vi "VarillaDataReadingStringToClusterFormar.vi"(11 "StringFormat":string[](array[string])) -> (3 "ClusterFormat":T1)   [LabVIEW 2014]
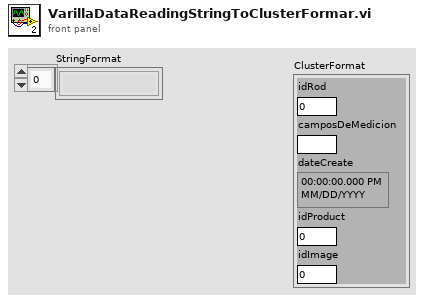
[diagram p1: front panel]
types:
  T1 = cluster{"idRod":dbl, "camposDeMedicion":string, "dateCreate":timestamp, "idProduct":dbl, "idImage":dbl}
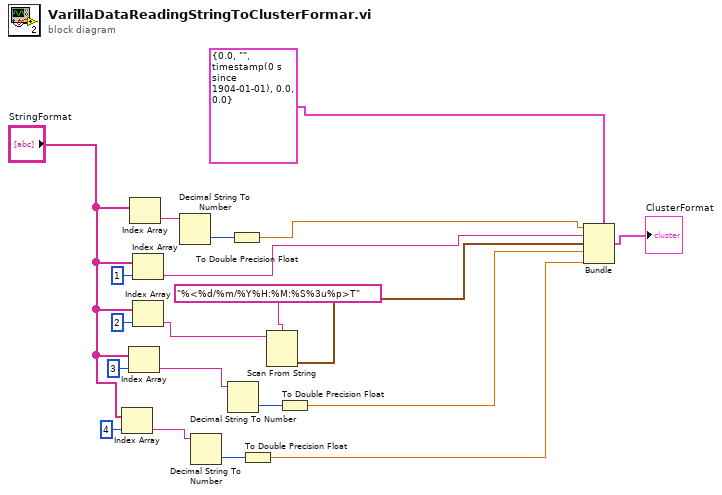
[diagram p0: block diagram]
diagram:
  n1 = Index Array(array="StringFormat", index=4) -> (element=w6:string)
  n2 = Index Array(array="StringFormat", index=3) -> (element=w9:string)
  n3 = Index Array(array="StringFormat") -> (element=w20:string)  [unwired: 1 in]
  n4 = Index Array(array="StringFormat", index=1) -> (element=w15:string)
  n5 = Index Array(array="StringFormat", index=2) -> (element=w3:string)
  n6 = Decimal String To Number(string=w20) -> (number=w17:i32)  [unwired: 2 in, 1 out]
  n7 = Decimal String To Number(string=w6) -> (number=w7:i32)  [unwired: 2 in, 1 out]
  n8 = Decimal String To Number(string=w9) -> (number=w10:i32)  [unwired: 2 in, 1 out]
  n9 = To Double Precision Float(number=w17) -> (double precision float=w16:dbl)
  n10 = To Double Precision Float(number=w7) -> (double precision float=w5:dbl)
  n11 = Scan From String(format string="%<%d/%m/%Y%H:%M:%S%3u%p>T", input string=w3) -> (output 1=w2:timestamp)  [unwired: 3 in, 3 out]
  n12 = To Double Precision Float(number=w10) -> (double precision float=w8:dbl)
  n13 = Bundle(cluster=T1 {"idRod"=0.0, "camposDeMedicion"="", "dateCreate"=timestamp(0 s since 1904-01-01), "idProduct"=0.0, "idImage"=0.0} ("Cluster of class private data"), "idRod"=w16, "camposDeMedicion"=w15, "dateCreate"=w2, "idProduct"=w8, "idImage"=w5) -> (→"ClusterFormat":T1)
